vi "Create Result.vi"(8 "error in (no error)":errorcluster, 11 "IV in":refnum<class "IV.lvclass">) -> (0 "error out":errorcluster, 2 "Text":string, 3 "IV out":refnum<class "IV.lvclass">)   [LabVIEW 2018, in "IV.lvclass"]
uses:
  IV.lvclass
  data/IV_data.lvclass
  Abstract/Data/Data2D/Data2D.lvclass
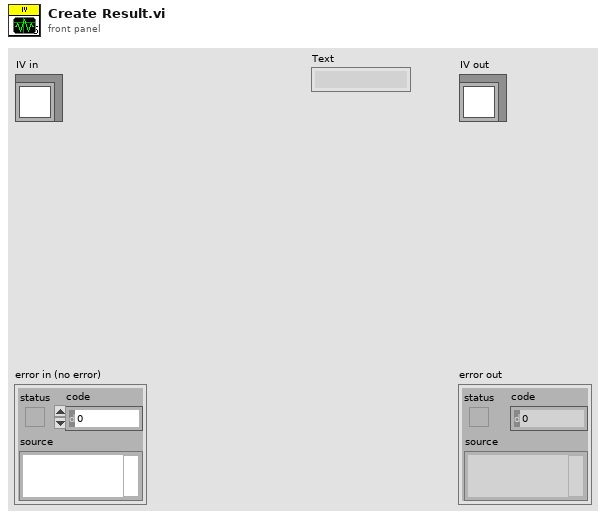
[diagram p1: front panel]
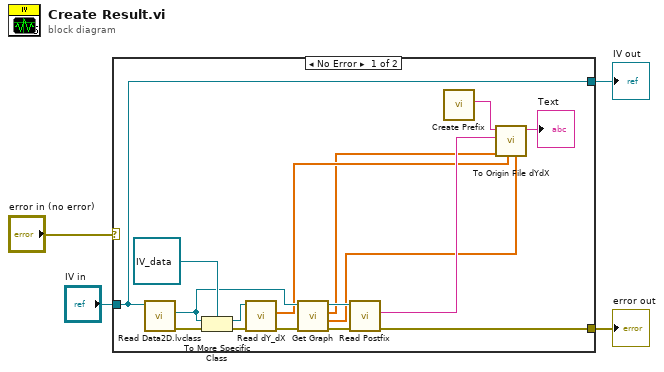
[diagram p0: block diagram]
diagram:
  n1 = case shown="No Error" "error in (no error)" {
    selector: "error in (no error)" -> [_ w22]
    tunnel: [w8 w22] -> w3
    tunnel: [w20 w21] -> w1
    tunnel: "IV in" -> [w20 w21]
    frame No Error {
      n2 = call-dynamic "Read Data2D.lvclass.vi"("Experiment2D in"=w20) -> ("error out"=w17:errorcluster, "Data2D.lvclass"=w15:refnum<class "Data2D.lvclass">)  [unwired: 8 in, 1 out]
      n3 = To More Specific Class(target class=refnum<class "IV_data.lvclass"> refnum ("IV_data.lvclass"), reference=w15, error in=w17) -> (specific class reference=w18:refnum<class "IV_data.lvclass">, error out=w16:errorcluster)
      n4 = call-dynamic "Read dY_dX.vi"("error in (no error)"=w16, "IV_data in"=w18) -> ("error out"=w9:errorcluster, "dY/dX"=w7:dbl[])  [unwired: 7 in, 1 out]
      n5 = call-dynamic "Get Graph.vi"("error in (no error)"=w9, "Data2D in"=w15) -> ("error out"=w10:errorcluster, "Y"=w5:dbl[], "X"=w6:dbl[], "Data2D out"=w12:refnum<class "Data2D.lvclass">)  [unwired: 6 in]
      n6 = call-dynamic "Read Postfix.vi"("error in (no error)"=w10, "Data2D in"=w12) -> ("error out"=w8:errorcluster, "Postfix"=w11:string)  [unwired: 7 in, 1 out]
      n7 = call "Create Prefix.vi"() -> ("Text"=w14:string)  [unwired: 11 in]
      n8 = call "To Origin File dYdX.vi"("Y"=w5, "dYdX"=w7, "X"=w6, "Postfix"=w11, "Prefix"=w14) -> ("Text"=→"Text":string)  [unwired: 6 in]
    }
    frame Error {
    }
  }
  "error out" <- w3
  "IV out" <- w1
